vi "beamModule.vi"() -> ()   [LabVIEW 2023, in "GUI.lvlib"]
uses:
  GUI.lvlib
panel:
  out "index":dbl
  out "beam0":cluster{dbl[], dbl[]}(graph)={[-0.6494, -0.65939, -0.5375, -0.58546, -0.55349, -0.63341, -0.63541, -0.73931, -1.5326, -1.7384, -1.6964, -1.7124, -2.3438, -2.198, -1.7104, -0.92714, -1.113, -1.7484, -1.3448, -1.097, -0.66738, -0.71534, -0.73332, -0.69536, -0.63341, -0.71534, -0.90316, -1.2888, -1.4926, -1.1829, -0.35167, -0.11989, 0.36566, 0.59345, 1.0071, 1.107, 0.70135, -0.5395, -1.9662, -2.5277, -2.4797, -3.247, -3.1171, -2.8154, -2.6096, -2.6116, -2.17, -2.0041, -2.0641, -2.2399, -2.6036, -2.4457, -2.106, -2.172, -1.6605, -1.6085, -1.7204, -2.176, -2.164, -1.1469, -0.81125, -1.8263, -1.2888, -1.3547, -1.027, -1.4007, -1.3128, -2.5177, -1.079, 0.84921, -2.6435, -2.2619, -2.8134, -3.191, -4.3759, -5.0493, -4.5778, -4.6777, -4.7776, -4.5198, -4.0642, -3.7845, -3.5287, -3.7006, -3.5807, -3.5147, -4.1282, -4.0423, -4.5578, -4.9814, -5.7067, -5.5449, -5.7487, -6.2102, -5.7547, -5.5089, -4.7396, -4.0502, -4.0223, -3.7785, -4.1182, -4.6197, -4.3699, -4.6457, -5.1193, -2.8973, -4.0323, -4.0443, -4.4079, -3.279, -3.0911], [0.0, 1.0, 2.0, 3.0, 4.0, 5.0, 6.0, 7.0, 8.0, 9.0, 10.0, 11.0, 12.0, 13.0, 14.0, 15.0, 16.0, 17.0, 18.0, 19.0, 20.0, 21.0, 22.0, 23.0, 24.0, 25.0, 26.0, 27.0, 28.0, 29.0, 30.0, 31.0, 32.0, 33.0, 34.0, 35.0, 36.0, 37.0, 38.0, 39.0, 40.0, 41.0, 42.0, 43.0, 44.0, 45.0, 46.0, 47.0, 48.0, 49.0, 50.0, 51.0, 52.0, 53.0, 54.0, 55.0, 56.0, 57.0, 58.0, 59.0, 60.0, 61.0, 62.0, 63.0, 64.0, 65.0, 66.0, 67.0, 68.0, 69.0, 70.0, 71.0, 72.0, 73.0, 74.0, 75.0, 76.0, 77.0, 78.0, 79.0, 80.0, 81.0, 82.0, 83.0, 84.0, 85.0, 86.0, 87.0, 88.0, 89.0, 90.0, 91.0, 92.0, 93.0, 94.0, 95.0, 96.0, 97.0, 98.0, 99.0, 100.0, 101.0, 102.0, 103.0, 104.0, 105.0, 106.0, 107.0, 108.0, 109.0, 110.0]}
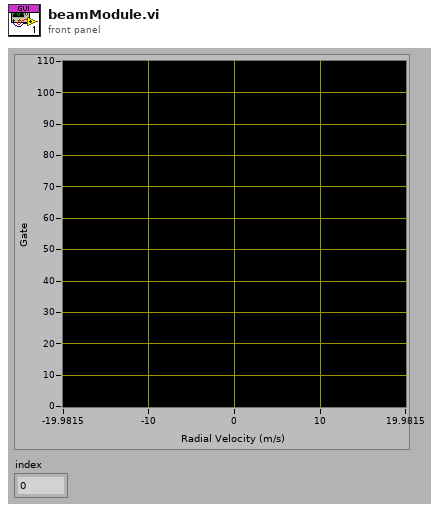
[diagram p1: front panel]
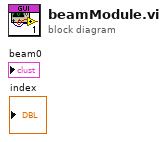
[diagram p0: block diagram]
diagram:
